vi "ModuleManager Page.vi"(8 "?":errorcluster) -> ()   [LabVIEW 2018, in "Vires VTD System Explorer.lvlib"]
uses:
  Vires VTD System Explorer.lvlib
  <vilib>/NI Veristand/Custom Device API/Custom Device Item Ref.ctl
  Shared/Sensor Name.ctl
  Shared/Protocol.ctl
  Shared/SensorInfo.ctl
  MM/MM Data.ctl
  MM/MM Objects.ctl
  MM/MM Object.ctl
  <vilib>/NI Veristand/Custom Device API/Custom Device API.lvlib
  Shared/Vires VTD Shared.lvlib
  MM/MM.lvlib
panel:
  in  "Tab Control":enum32{"Sensor"}(tab)
  in  "PlayerID":u8=1
  in  "Add Sensor":bool
  in  "# Culled Objects":i32=1
  in  "Network port":i32=48185
  in  "Protocol":T1
  in  "Sensor Name":T2
  in  "Header":cluster{"Section Name":string}={"Section Name"="Custom Device Item Settings"}
  in  "Description":string
  in  "Name":string
  in  "Node Ptr":T3 format="%.0x"
  out "error out":errorcluster
  in  "SHDocVw.IWebBrowser2":refnum<k7>(container)
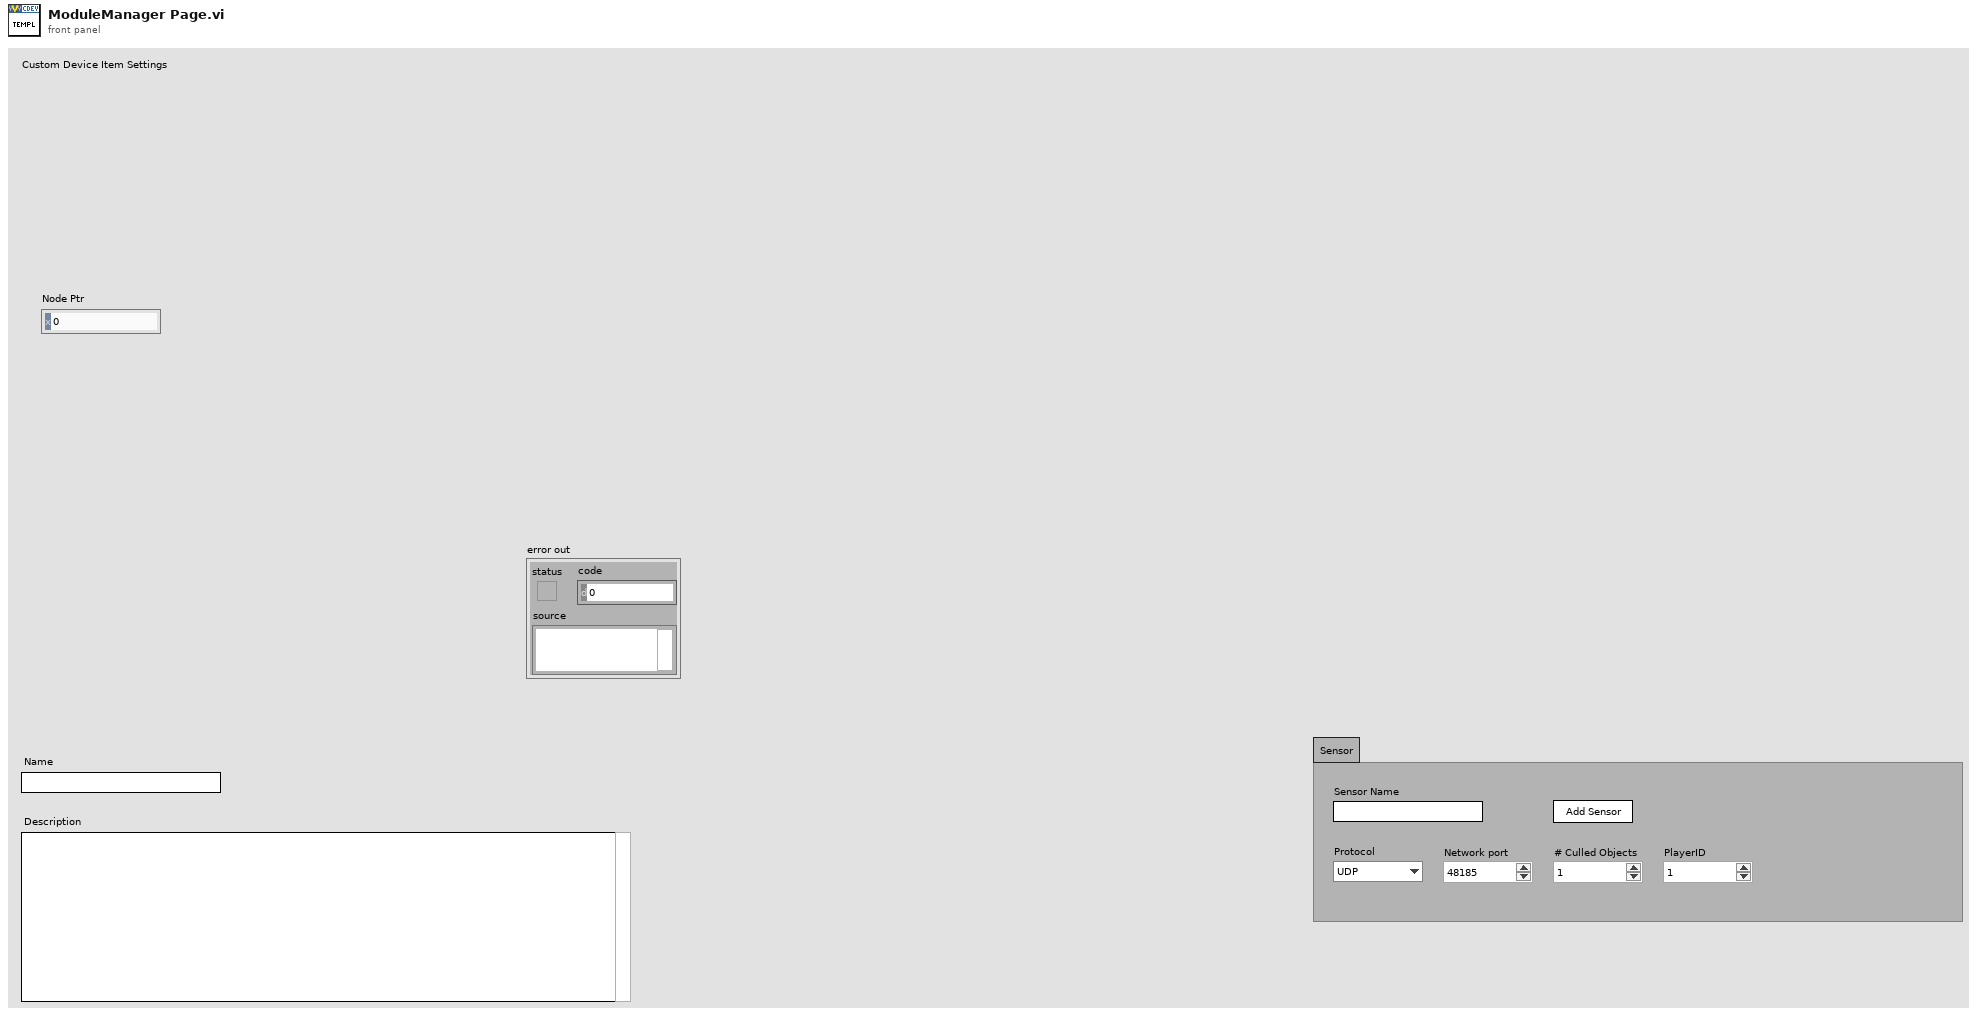
[diagram p1: front panel]
types:
  T1 = typedef "Vires VTD Shared.lvlib/Protocol.ctl" = enum16{"UDP", "TCP"}
  T2 = typedef "Vires VTD Shared.lvlib/Sensor Name.ctl" = string
  T3 = typedef "Custom Device API.lvlib/Custom Device Item Ref.ctl" = u64
  T4 = typedef "Custom Device API.lvlib/Custom Device Item Info.ctl" = cluster{"Name":string, "Is Channel":bool, "GUID":string, "Is Waveform":bool}
  T5 = typedef "Vires VTD Shared.lvlib/SensorInfo.ctl" = cluster{"Sensor Name":T2, "Protocol":T1, "Network port":i32, "# Culled Objects":i32, "PlayerID":u8, "MM Data":T6}
  T6 = typedef "Vires VTD Shared.lvlib/MM Data.ctl" = T7[]
  T7 = typedef "MM.lvlib/MM Objects.ctl" = cluster{"pkID":i32, "MM Objects":T8[]}
  T8 = typedef "MM.lvlib/MM Object.ctl" = cluster{"Object":i32, "Signals":string[]}
  T9 = typedef "Custom Device API.lvlib/Custom Device Commands.ctl" = enum16{"Default", "Item renamed", "Shutdown", "Dynamic button pressed"}
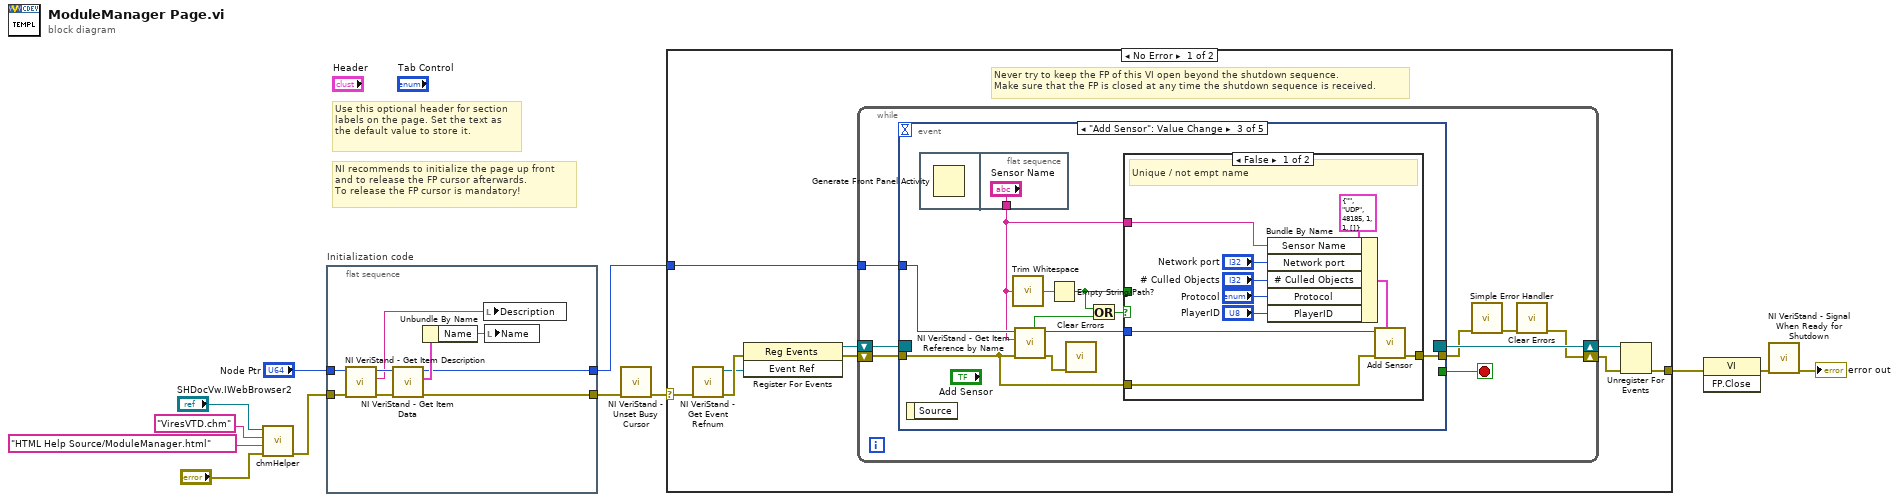
[diagram p0: block diagram]
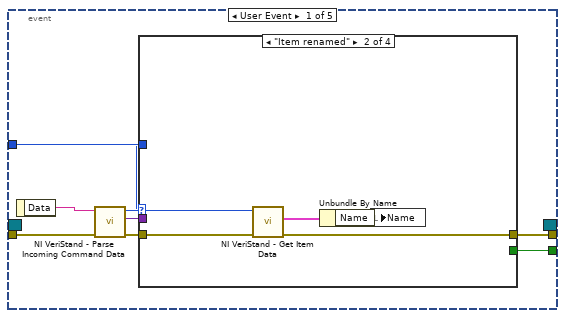
[diagram p2: hidden frame]
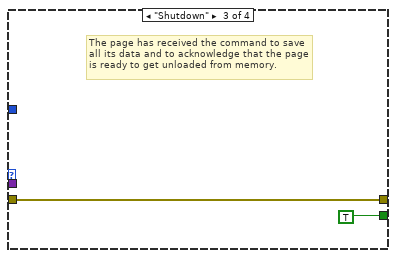
[diagram p4: hidden frame]
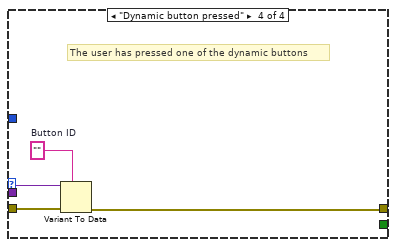
[diagram p5: hidden frame]
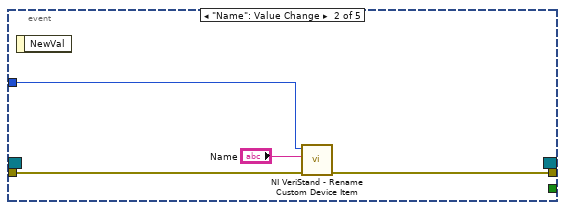
[diagram p6: hidden frame]
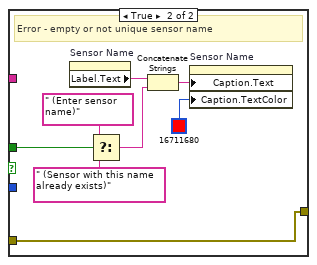
[diagram p7: hidden frame]
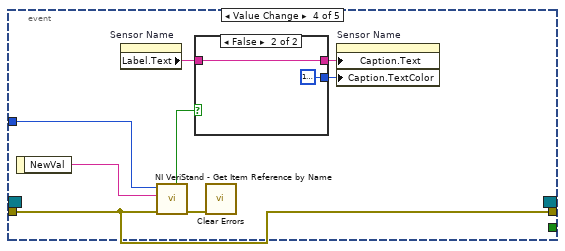
[diagram p8: hidden frame]
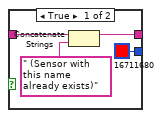
[diagram p9: hidden frame]
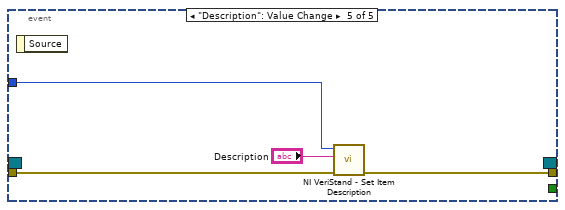
[diagram p10: hidden frame]
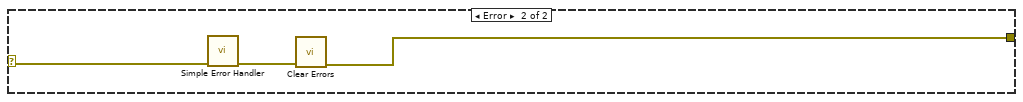
[diagram p11: hidden frame]
diagram:
  # "Use this optional header for section labels on the page. Set the text as the default value to store it."
  # "NI recommends to initialize the page up front\nand to release the FP cursor afterwards.\nTo release the FP cursor is mandatory!"
  n1 = call "chmHelper.vi"("error in (no error)"="?", "HTML File"="HTML Help Source/ModuleManager.html", "Main CHM File"="ViresVTD.chm" ("HTML File"), "Automation Refnum in"="SHDocVw.IWebBrowser2") -> ("error out"=w2:errorcluster)  [unwired: 7 in]
  n2 = flat-sequence "Initialization code" {
    tunnel: w2 -> [w20]
    tunnel: "Node Ptr" -> [w19]
    tunnel: [w15] -> w4
    tunnel: [w16] -> w1
    frame #0 {
      n3 = call <vilib>:"NI VeriStand - Get Item Description.vi"("error in (no error)"=w20, "Item Ref in"=w19) -> ("error out"=w18:errorcluster, "Description"=w14:string, "Item Ref out"=w21:T3)  [unwired: 7 out]
      n4 = call <vilib>:"NI VeriStand - Get Item Data.vi"("error in (no error)"=w18, "Item Ref in"=w21) -> ("error out"=w15:errorcluster, "Item Info"=w17:T4, "Item Ref out"=w16:T3)  [unwired: 7 out]
      n5 = Unbundle By Name(w17) -> ("Name"=w13:string)
      n6 = local write "Description"(w14) -> ()
      n7 = local write "Name"(w13) -> ()
    }
  }
  n8 = call <vilib>:"NI VeriStand - Unset Busy Cursor.vi"("error in (no error)"=w4) -> ("error out"=w3:errorcluster)  [unwired: 10 out]
  n9 = case shown="No Error" w3 {
    selector: w3 -> [w22 w112]
    tunnel: [w27 w110] -> w8
    tunnel: w1 -> [w23 _]
    frame No Error {
      # "Never try to keep the FP of this VI open beyond the shutdown sequence.\nMake sure that the FP is closed at any time the shutdown sequence is received."
      n10 = call <vilib>:"NI VeriStand - Get Event Refnum.vi"("error in (no error)"=w22) -> ("error out"=w30:errorcluster, "Event Ref"=w26:refnum<user-event>)  [unwired: 9 out]
      n11 = register-events(error in=w30, w26) -> (reference out=w24:refnum<event-registration>, error out=w25:errorcluster)  [unwired: 1 in]
      n12 = while {
        tunnel: w23 -> [w34]
        shift-right: [w31] -> w28
        shift-left: w25 -> [w37]
        shift-right: [w38] -> w29
        shift-left: w24 -> [w36]
        stop <- w35 stop-if-true
        n13 = event shown="[2] \"Add Sensor\": Value Change" {
          selector: w36 -> [_ _ _ _ _]
          dyn-events: [_ _ _ _ _] -> w38
          timeout: _ -> [_ _ _ _ _]
          tunnel: w37 -> [w46 w62 w65 w93 w108]
          tunnel: [w42 _ _ _ _] -> w35
          tunnel: [w41 w61 w72 w93 w107] -> w33
          tunnel: w34 -> [w40 w60 w71 w99 w109]
          event User Event {
            n14 = event-data() -> ("Data"=w45:string)  [unwired: 1 out]
            n15 = call <vilib>:"NI VeriStand - Parse Incoming Command Data.vi"("error in (no error)"=w46, "Incoming data"=w45) -> ("error out"=w44:errorcluster, "Outgoing data"=w39:variant, "Action"=w43:T9)  [unwired: 7 out]
            n16 = case shown="\"Item renamed\"" w43 {
              tunnel: w44 -> [w47 w52 w53 w58]
              tunnel: [_ _ TRUE _] -> w42
              tunnel: [w47 w50 w53 w55] -> w41
              tunnel: w40 -> [_ w48 _ _]
              tunnel: w39 -> [_ _ _ w57]
              frame "Default", Default {
              }
              frame "Item renamed" {
                n17 = call <vilib>:"NI VeriStand - Get Item Data.vi"("error in (no error)"=w52, "Item Ref in"=w48) -> ("error out"=w50:errorcluster, "Item Info"=w51:T4)  [unwired: 8 out]
                n18 = Unbundle By Name(w51) -> ("Name"=w49:string)
                n19 = local write "Name"(w49) -> ()
              }
              frame "Shutdown" {
                # "The page has received the command to save all its data and to acknowledge that the page is ready to get unloaded from memory."
              }
              frame "Dynamic button pressed" {
                w56 = ""  # Button ID
                # "The user has pressed one of the dynamic buttons"
                n20 = Variant To Data(error in=w58, type=w56, Variant=w57) -> (error out=w55:errorcluster)  [unwired: 1 out]
              }
            }
          }
          event "Name": Value Change {
            n21 = event-data() -> ()  [unwired: 2 out]
            n22 = call <vilib>:"NI VeriStand - Rename Custom Device Item.vi"("error in (no error)"=w62, "New Name"="Name", "Item Ref in"=w60) -> ("error out"=w61:errorcluster)  [unwired: 1 in, 7 out]
          }
          event "Add Sensor": Value Change {
            n23 = event-data() -> ()  [unwired: 2 out]
            n24 = flat-sequence {
              tunnel: ["Sensor Name"] -> w63
              frame #0 {
                n25 = Generate Front Panel Activity() -> ()  [unwired: 1 in]
              }
              frame #1 {
              }
            }
            n26 = call <vilib>:"Trim Whitespace.vi"("string"=w63) -> ("trimmed string"=w68:string)  [unwired: 1 in]
            n27 = call <vilib>:"NI VeriStand - Get Item Reference by Name.vi"("error in (no error)"=w65, "Item Name"=w63, "Parent Ref in"=w71) -> ("error out"=w64:errorcluster, "Parent Ref out"=w70:T3, "Found"=w69:bool)  [unwired: 5 in, 1 out]
            n28 = Empty String/Path?(string/path=w68) -> (empty?=w66:bool)
            n29 = call <vilib>:"Clear Errors.vi"("error in (no error)"=w64) -> ()  [unwired: 1 in, 6 out]
            n30 = Or(x=w66, y=w69) -> (x .or. y?=w67:bool)
            n31 = case shown="False" w67 {
              tunnel: [w83 w84] -> w72
              tunnel: w70 -> [w82 _]
              tunnel: w63 -> [w75 _]
              tunnel: w66 -> [_ w85]
              tunnel: w65 -> [w74 w84]
              frame False {
                # "Unique / not empt name"
                n32 = Bundle By Name(cluster=T5 {"Sensor Name"="", "Protocol"=enum."UDP", "Network port"=48185, "# Culled Objects"=1, "PlayerID"=1, "MM Data"=[]} ("SensorInfo"), "Sensor Name"=w75, "Network port"="Network port", "# Culled Objects"="# Culled Objects", "Protocol"="Protocol", "PlayerID"="PlayerID") -> (w76:T5)
                n33 = call "Add Sensor.vi"("SensorInfo"=w76, "error in (no error)"=w74, "Item Ref in"=w82) -> ("error out (no error)"=w83:errorcluster)  [unwired: 8 in]
              }
              frame True {
                # "Error - empty or not unique sensor name"
                n34 = property on="Sensor Name" class="Str (strict)"() -> ("Label.Text"=w90:string)  [unwired: 2 in, 2 out]
                n35 = Select(t=" (Enter sensor name)" ("string"), s=w85, f=" (Sensor with this name already exists)" ("string")) -> (s? t:f=w88:string)
                n36 = Concatenate Strings(w90, w88) -> (w91:string)
                n37 = property on="Sensor Name" class="Str (strict)"("Caption.Text"=w91, "Caption.TextColor"=u32 16711680) -> ()  [unwired: 2 in, 2 out]
              }
            }
          }
          event Value Change {
            n38 = event-data() -> ("NewVal"=w98:T2)  [unwired: 1 out]
            n39 = property on="Sensor Name" class="Str (strict)"() -> ("Label.Text"=w95:string)  [unwired: 2 in, 2 out]
            n40 = call <vilib>:"NI VeriStand - Get Item Reference by Name.vi"("error in (no error)"=w93, "Item Name"=w98, "Parent Ref in"=w99) -> ("error out"=w92:errorcluster, "Found"=w97:bool)  [unwired: 5 in, 2 out]
            n41 = case shown="False" w97 {
              tunnel: [u32 16711680 u32 16777222] -> w94
              tunnel: [w101 w104] -> w96
              tunnel: w95 -> [w102 w104]
              frame True {
                n42 = Concatenate Strings(w102, " (Sensor with this name already exists)" ("string")) -> (w101:string)
              }
              frame False {
              }
            }
            n43 = call <vilib>:"Clear Errors.vi"("error in (no error)"=w92) -> ()  [unwired: 1 in, 6 out]
            n44 = property on="Sensor Name" class="Str (strict)"("Caption.Text"=w96, "Caption.TextColor"=w94) -> ()  [unwired: 2 in, 2 out]
          }
          event "Description": Value Change {
            n45 = event-data() -> ()  [unwired: 2 out]
            n46 = call <vilib>:"NI VeriStand - Set Item Description.vi"("error in (no error)"=w108, "Description"="Description", "Item Ref in"=w109) -> ("error out"=w107:errorcluster)  [unwired: 8 out]
          }
        }
        n47 = call <vilib>:"Simple Error Handler.vi"("error in (no error)"=w33) -> ("error out"=w32:errorcluster)  [unwired: 1 in, 7 out]
        n48 = call <vilib>:"Clear Errors.vi"("error in (no error)"=w32) -> ("error out"=w31:errorcluster)  [unwired: 1 in, 5 out]
      }
      n49 = Unregister For Events(event registration refnum=w29, error in=w28) -> (error out=w27:errorcluster)
    }
    frame Error {
      n50 = call <vilib>:"Simple Error Handler.vi"("error in (no error)"=w112) -> ("error out"=w111:errorcluster)  [unwired: 1 in, 7 out]
      n51 = call <vilib>:"Clear Errors.vi"("error in (no error)"=w111) -> ("error out"=w110:errorcluster)  [unwired: 1 in, 5 out]
    }
  }
  n52 = invoke class="VI" method="FP.Close"(error in=w8) -> (error out=w7:errorcluster)  [unwired: 2 in, 2 out]
  n53 = call <vilib>:"NI VeriStand - Signal When Ready for Shutdown.vi"("error in (no error)"=w7) -> ("error out"=→"error out":errorcluster)  [unwired: 10 out]
